vi "Read Left Power.vi"(8 "error in (no error)":errorcluster, 11 "Drive Continuous Cmd in":refnum<class "Drive by Power.lvclass">) -> (0 "error out":errorcluster, 2 "Left Power":dbl min=-1.0 max=1.0, 3 "Drive Continuous Cmd out":refnum<class "Drive by Power.lvclass">)   [LabVIEW 2014, in "Forward Drive.lvlib" / "Drive by Power.lvclass"]
uses:
  Drive by Power.lvclass
  Drive by Power.lvclass/Drive by Power.ctl
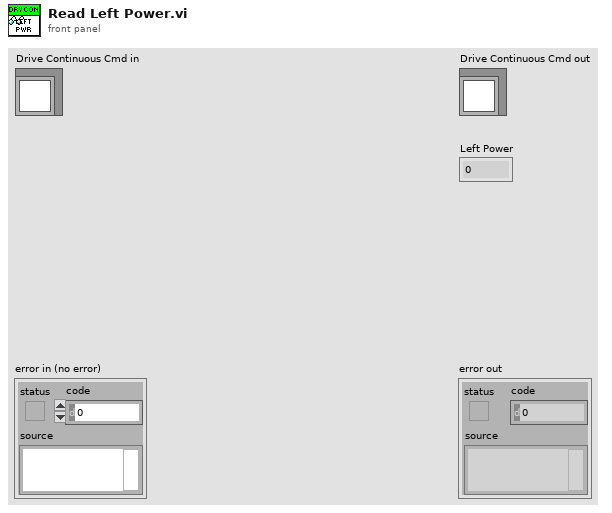
[diagram p1: front panel]
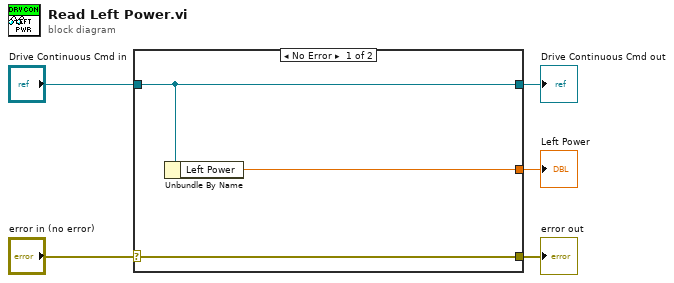
[diagram p0: block diagram]
diagram:
  n1 = case shown="No Error" "error in (no error)" {
    selector: "error in (no error)" -> [w8 w9]
    tunnel: [w8 w9] -> w4
    tunnel: [w7 w10] -> w2
    tunnel: "Drive Continuous Cmd in" -> [w7 w10]
    tunnel: [w6 _] -> w1
    frame No Error {
      n2 = Unbundle By Name(w7) -> ("Left Power"=w6:dbl)
    }
    frame Error {
    }
  }
  "error out" <- w4
  "Drive Continuous Cmd out" <- w2
  "Left Power" <- w1
